vi "XIPIN_3GPP_LTE_MIMO_Decoder_2_0.vi"   [LabVIEW 2017]
doc: "The 3GPP LTE MIMO Decoder LogiCORE is a drop-in module for Virtex-5(TM), Virtex-6(TM) and Virtex-6L(TM) families of FPGA. It performs MIMO decoding using the MMSE algorithm. The core is fully synchronous, using a single clock, and integrates seamlessly with the Xilinx design flow.\n------------------------------------\n<b>Need License</b> : Yes\n<b>Interface</b> : AXI_STREAMING"
uses:
  <vilib>/rvi/XilinxIP/XIPIN_XNode/niFpgaXIPIN.xnode
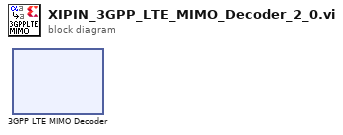
[diagram p0: block diagram]
diagram:
  n1 = xnode ("3GPP LTE MIMO Decoder")() -> ()
